vi "Take Snapshot.vi"(8 "error in":errorcluster, 11 "Electronic Load in":refnum<class "Electronic Load.lvclass">) -> (0 "error out":errorcluster, 3 "Electronic Load out":refnum<class "Electronic Load.lvclass">)   [LabVIEW 2019, in "Electronic Load.lvlib" / "Electronic Load.lvclass"]
doc: "Use Snapshot Data to Generate a Group Separated Snapshot record. This eliminates nearly all the overhead in creating and removing a record group for snapshot data."
uses:
  Library/Electronic Load.lvclass
  builds/Instruments/Instruments.lvlibp/Library/Instruments.lvclass
  C:/Users/Public/Documents/Development/builds/Instruments/Instruments.lvlibp/Library/Instruments.lvclass
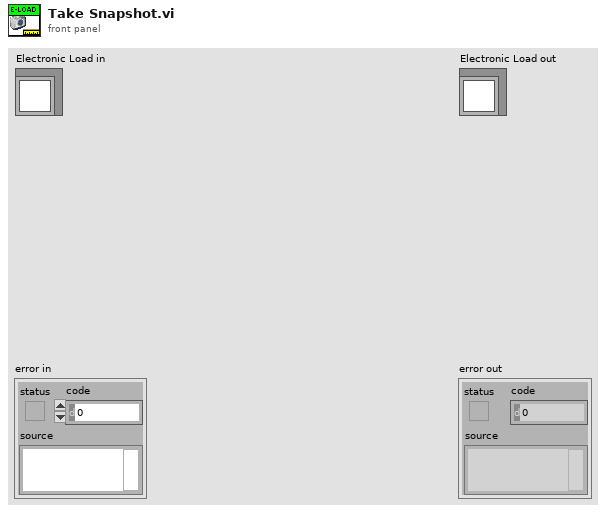
[diagram p1: front panel]
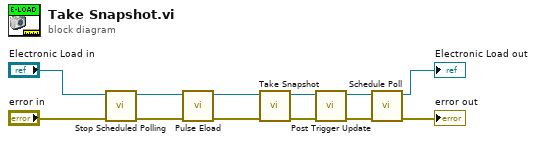
[diagram p0: block diagram]
diagram:
  n1 = call "Stop Scheduled Polling.vi"("error in"="error in", "Instruments in"="Electronic Load in") -> ("error out"=w8:errorcluster, "Instruments out"=w7:refnum<class "Electronic Load.lvclass">)  [unwired: 8 in]
  n2 = call "Pulse Eload.vi"("error in"=w8, "Electronic Load in"=w7) -> ("error out"=w5:errorcluster, "Electronic Load out"=w6:refnum<class "Electronic Load.lvclass">)  [unwired: 8 in]
  n3 = call-parent "Take Snapshot.vi"("error in"=w5, "Instruments in"=w6) -> ("error out"=w3:errorcluster, "Instruments out"=w4:refnum<class "Electronic Load.lvclass">)  [unwired: 8 in]
  n4 = call "Post Trigger Update.vi"("error in"=w3, "Electronic Load in"=w4) -> ("error out"=w2:errorcluster, "Electronic Load out"=w1:refnum<class "Electronic Load.lvclass">)  [unwired: 8 in]
  n5 = call "Schedule Poll.vi"("error in"=w2, "Instruments in"=w1) -> ("error out"=→"error out":errorcluster, "Instruments out"=→"Electronic Load out":refnum<class "Electronic Load.lvclass">)  [unwired: 8 in]
